vi "DO.vi"(8 "error in (no error)":errorcluster, 10 "数据输出":T1, 11 "功能编号":u16(ring)) -> (0 "error out":errorcluster)   [LabVIEW 2017]
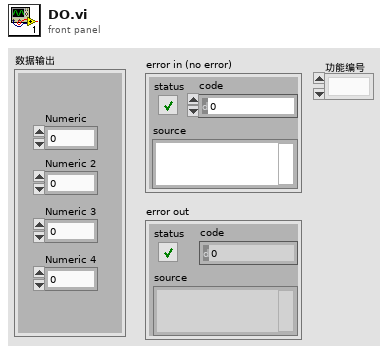
[diagram p1: front panel]
types:
  T1 = cluster{"Numeric":dbl, "Numeric 2":dbl, "Numeric 3":dbl, "Numeric 4":dbl}
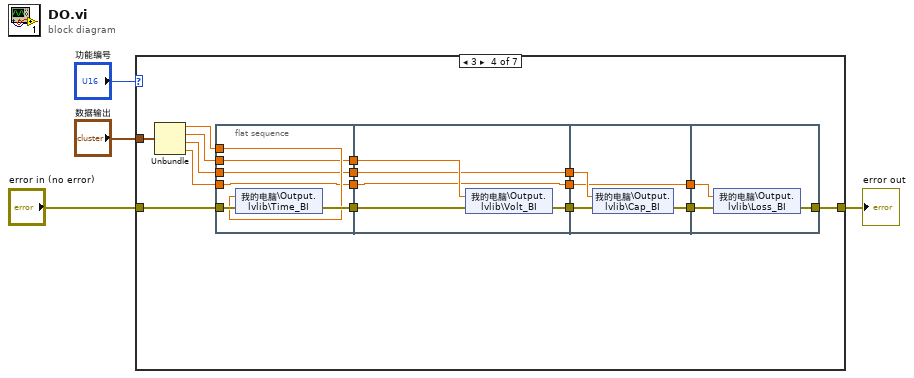
[diagram p0: block diagram]
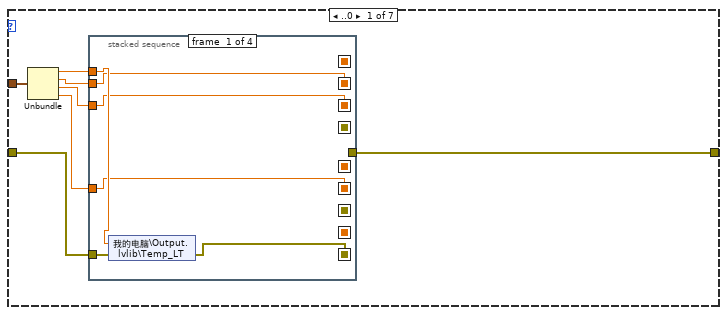
[diagram p2: hidden frame]
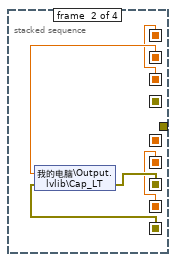
[diagram p3: hidden frame]
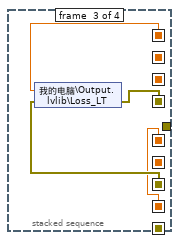
[diagram p4: hidden frame]
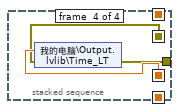
[diagram p5: hidden frame]
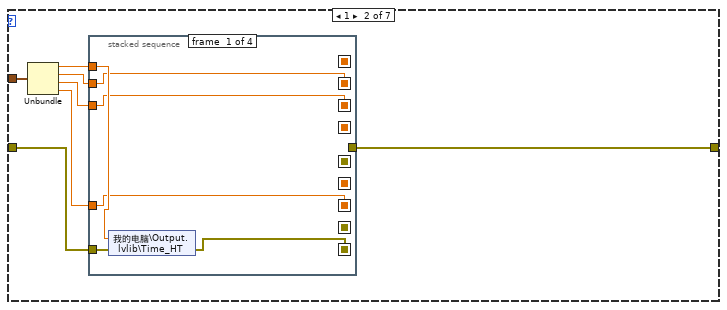
[diagram p6: hidden frame]
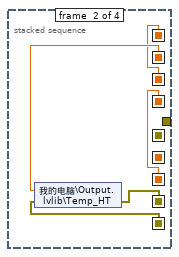
[diagram p7: hidden frame]
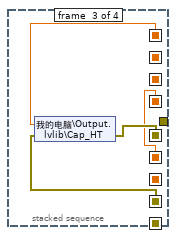
[diagram p8: hidden frame]
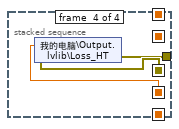
[diagram p9: hidden frame]
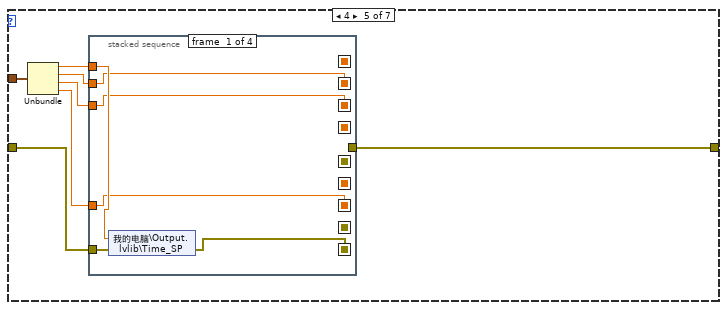
[diagram p11: hidden frame]
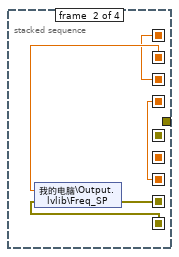
[diagram p12: hidden frame]
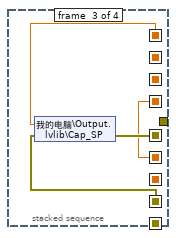
[diagram p13: hidden frame]
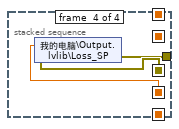
[diagram p14: hidden frame]
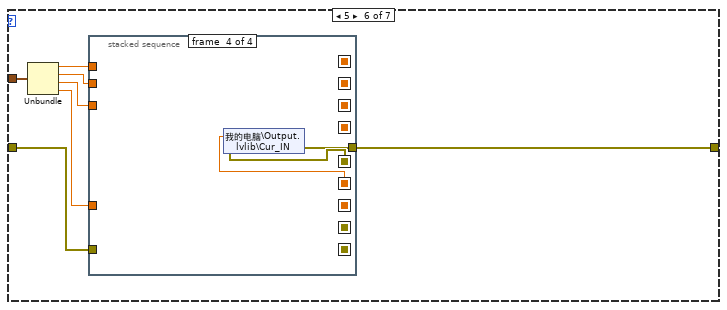
[diagram p15: hidden frame]
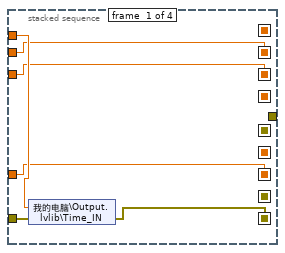
[diagram p16: hidden frame]
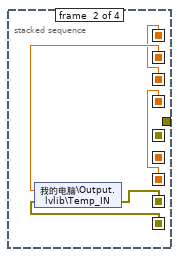
[diagram p17: hidden frame]
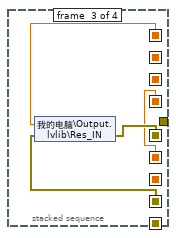
[diagram p18: hidden frame]
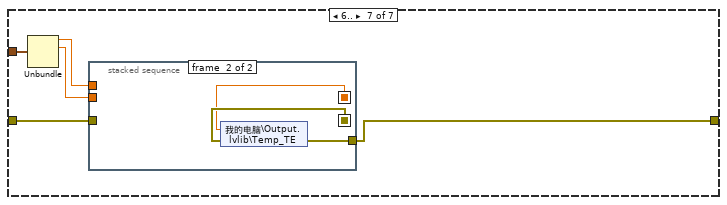
[diagram p19: hidden frame]
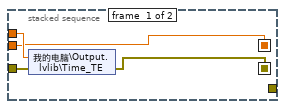
[diagram p20: hidden frame]
diagram:
  n1 = case shown="3" "功能编号" {
    tunnel: "数据输出" -> [w11 w36 _ w69 w96 w121 w142]
    tunnel: "error in (no error)" -> [w6 w35 w55 w71 w95 w120 w144]
    tunnel: [w5 w34 w55 w70 w94 w119 w143] -> w2
    frame ..0 {
      n2 = Unbundle(w11) -> ("Numeric"=w10:dbl, "Numeric 2"=w9:dbl, "Numeric 3"=w8:dbl, "Numeric 4"=w7:dbl)
      n3 = stacked-sequence {
        seq-local: [w14 _ _ _] -> [_ w22 _ _]
        seq-local: [w13 _ _ _] -> [_ w19 _ _]
        seq-local: [w12 _ _ _] -> [_ w18 _ _]
        seq-local: [w15 _ _ _] -> [_ w21 _ _]
        seq-local: [_ w19 _ _] -> [_ _ w26 _]
        seq-local: [_ w18 _ _] -> [_ _ w23 _]
        seq-local: [_ w20 _ _] -> [_ _ w25 _]
        seq-local: [_ _ w23 _] -> [_ _ _ w29]
        seq-local: [_ _ w24 _] -> [_ _ _ w28]
        tunnel: w10 -> [w17 _ _ _]
        tunnel: w6 -> [w16 _ _ _]
        tunnel: w9 -> [w14 _ _ _]
        tunnel: w8 -> [w13 _ _ _]
        tunnel: w7 -> [w12 _ _ _]
        tunnel: [_ _ _ w27] -> w5
        frame #0 {
          n4 = shared-variable "我的电脑\\Output.lvlib\\Temp_LT"(w17, error in=w16) -> (error out=w15:errorcluster)
        }
        frame #1 {
          n5 = shared-variable "我的电脑\\Output.lvlib\\Cap_LT"(w22, error in=w21) -> (error out=w20:errorcluster)
        }
        frame #2 {
          n6 = shared-variable "我的电脑\\Output.lvlib\\Loss_LT"(w26, error in=w25) -> (error out=w24:errorcluster)
        }
        frame #3 {
          n7 = shared-variable "我的电脑\\Output.lvlib\\Time_LT"(w29, error in=w28) -> (error out=w27:errorcluster)
        }
      }
    }
    frame 1 {
      n8 = Unbundle(w36) -> ("Numeric"=w33:dbl, "Numeric 2"=w32:dbl, "Numeric 3"=w31:dbl, "Numeric 4"=w30:dbl)
      n9 = stacked-sequence {
        seq-local: [w41 _ _ _] -> [_ w47 _ _]
        seq-local: [w39 _ _ _] -> [_ w45 _ _]
        seq-local: [w38 _ _ _] -> [_ w44 _ _]
        seq-local: [w37 _ _ _] -> [_ w43 _ _]
        seq-local: [_ w46 _ _] -> [_ _ w51 _]
        seq-local: [_ w44 _ _] -> [_ _ w49 _]
        seq-local: [_ w43 _ _] -> [_ _ w48 _]
        seq-local: [_ _ w50 _] -> [_ _ _ w54]
        seq-local: [_ _ w48 _] -> [_ _ _ w52]
        tunnel: w35 -> [w42 _ _ _]
        tunnel: w33 -> [w40 _ _ _]
        tunnel: w32 -> [w39 _ _ _]
        tunnel: w31 -> [w38 _ _ _]
        tunnel: w30 -> [w37 _ _ _]
        tunnel: [_ _ _ w53] -> w34
        frame #0 {
          n10 = shared-variable "我的电脑\\Output.lvlib\\Time_HT"(w40, error in=w42) -> (error out=w41:errorcluster)
        }
        frame #1 {
          n11 = shared-variable "我的电脑\\Output.lvlib\\Temp_HT"(w45, error in=w47) -> (error out=w46:errorcluster)
        }
        frame #2 {
          n12 = shared-variable "我的电脑\\Output.lvlib\\Cap_HT"(w49, error in=w51) -> (error out=w50:errorcluster)
        }
        frame #3 {
          n13 = shared-variable "我的电脑\\Output.lvlib\\Loss_HT"(w52, error in=w54) -> (error out=w53:errorcluster)
        }
      }
    }
    frame 2 {
    }
    frame 3 {
      n14 = Unbundle(w69) -> ("Numeric"=w68:dbl, "Numeric 2"=w67:dbl, "Numeric 3"=w66:dbl, "Numeric 4"=w65:dbl)
      n15 = flat-sequence {
        tunnel: w71 -> [w77]
        tunnel: w68 -> [w75]
        tunnel: w67 -> [w74]
        tunnel: w66 -> [w73]
        tunnel: w65 -> [w72]
        tunnel: [w76] -> w64
        tunnel: [w74] -> w63
        tunnel: [w73] -> w62
        tunnel: [w72] -> w61
        tunnel: w64 -> [w82]
        tunnel: w63 -> [w80]
        tunnel: w62 -> [w79]
        tunnel: w61 -> [w78]
        tunnel: [w81] -> w60
        tunnel: [w79] -> w59
        tunnel: [w78] -> w58
        tunnel: w60 -> [w86]
        tunnel: w59 -> [w84]
        tunnel: w58 -> [w83]
        tunnel: [w85] -> w57
        tunnel: [w83] -> w56
        tunnel: [w88] -> w70
        tunnel: w57 -> [w89]
        tunnel: w56 -> [w87]
        frame #0 {
          n16 = shared-variable "我的电脑\\Output.lvlib\\Time_BI"(w75, error in=w77) -> (error out=w76:errorcluster)
        }
        frame #1 {
          n17 = shared-variable "我的电脑\\Output.lvlib\\Volt_BI"(w80, error in=w82) -> (error out=w81:errorcluster)
        }
        frame #2 {
          n18 = shared-variable "我的电脑\\Output.lvlib\\Cap_BI"(w84, error in=w86) -> (error out=w85:errorcluster)
        }
        frame #3 {
          n19 = shared-variable "我的电脑\\Output.lvlib\\Loss_BI"(w87, error in=w89) -> (error out=w88:errorcluster)
        }
      }
    }
    frame 4 {
      n20 = Unbundle(w96) -> ("Numeric"=w93:dbl, "Numeric 2"=w92:dbl, "Numeric 3"=w91:dbl, "Numeric 4"=w90:dbl)
      n21 = stacked-sequence {
        seq-local: [w101 _ _ _] -> [_ w107 _ _]
        seq-local: [w99 _ _ _] -> [_ w105 _ _]
        seq-local: [w98 _ _ _] -> [_ w104 _ _]
        seq-local: [w97 _ _ _] -> [_ w103 _ _]
        seq-local: [_ w106 _ _] -> [_ _ w111 _]
        seq-local: [_ w104 _ _] -> [_ _ w109 _]
        seq-local: [_ w103 _ _] -> [_ _ w108 _]
        seq-local: [_ _ w110 _] -> [_ _ _ w114]
        seq-local: [_ _ w108 _] -> [_ _ _ w112]
        tunnel: w95 -> [w102 _ _ _]
        tunnel: w93 -> [w100 _ _ _]
        tunnel: w92 -> [w99 _ _ _]
        tunnel: w91 -> [w98 _ _ _]
        tunnel: w90 -> [w97 _ _ _]
        tunnel: [_ _ _ w113] -> w94
        frame #0 {
          n22 = shared-variable "我的电脑\\Output.lvlib\\Time_SP"(w100, error in=w102) -> (error out=w101:errorcluster)
        }
        frame #1 {
          n23 = shared-variable "我的电脑\\Output.lvlib\\Freq_SP"(w105, error in=w107) -> (error out=w106:errorcluster)
        }
        frame #2 {
          n24 = shared-variable "我的电脑\\Output.lvlib\\Cap_SP"(w109, error in=w111) -> (error out=w110:errorcluster)
        }
        frame #3 {
          n25 = shared-variable "我的电脑\\Output.lvlib\\Loss_SP"(w112, error in=w114) -> (error out=w113:errorcluster)
        }
      }
    }
    frame 5 {
      n26 = Unbundle(w121) -> ("Numeric"=w118:dbl, "Numeric 2"=w117:dbl, "Numeric 3"=w116:dbl, "Numeric 4"=w115:dbl)
      n27 = stacked-sequence {
        seq-local: [w126 _ _ _] -> [_ w132 _ _]
        seq-local: [w124 _ _ _] -> [_ w130 _ _]
        seq-local: [w123 _ _ _] -> [_ w129 _ _]
        seq-local: [w122 _ _ _] -> [_ w128 _ _]
        seq-local: [_ w131 _ _] -> [_ _ w136 _]
        seq-local: [_ w129 _ _] -> [_ _ w134 _]
        seq-local: [_ w128 _ _] -> [_ _ w133 _]
        seq-local: [_ _ w135 _] -> [_ _ _ w139]
        seq-local: [_ _ w133 _] -> [_ _ _ w137]
        tunnel: w120 -> [w127 _ _ _]
        tunnel: w118 -> [w125 _ _ _]
        tunnel: w117 -> [w124 _ _ _]
        tunnel: w116 -> [w123 _ _ _]
        tunnel: w115 -> [w122 _ _ _]
        tunnel: [_ _ _ w138] -> w119
        frame #0 {
          n28 = shared-variable "我的电脑\\Output.lvlib\\Time_IN"(w125, error in=w127) -> (error out=w126:errorcluster)
        }
        frame #1 {
          n29 = shared-variable "我的电脑\\Output.lvlib\\Temp_IN"(w130, error in=w132) -> (error out=w131:errorcluster)
        }
        frame #2 {
          n30 = shared-variable "我的电脑\\Output.lvlib\\Res_IN"(w134, error in=w136) -> (error out=w135:errorcluster)
        }
        frame #3 {
          n31 = shared-variable "我的电脑\\Output.lvlib\\Cur_IN"(w137, error in=w139) -> (error out=w138:errorcluster)
        }
      }
    }
    frame 6.. {
      n32 = Unbundle(w142) -> ("Numeric"=w141:dbl, "Numeric 2"=w140:dbl)  [unwired: 2 out]
      n33 = stacked-sequence {
        seq-local: [w147 _] -> [_ w151]
        seq-local: [w145 _] -> [_ w149]
        tunnel: w144 -> [w148 _]
        tunnel: w141 -> [w146 _]
        tunnel: w140 -> [w145 _]
        tunnel: [_ w150] -> w143
        frame #0 {
          n34 = shared-variable "我的电脑\\Output.lvlib\\Time_TE"(w146, error in=w148) -> (error out=w147:errorcluster)
        }
        frame #1 {
          n35 = shared-variable "我的电脑\\Output.lvlib\\Temp_TE"(w149, error in=w151) -> (error out=w150:errorcluster)
        }
      }
    }
  }
  "error out" <- w2
